vi "GetActionEventValue.vi"(8 "error in (no error)":errorcluster, 10 "Action":T1, 11 "WindowFrame in":refnum<class "WindowFrame.lvclass">) -> (0 "error out":errorcluster, 2 "Variant":variant, 3 "WindowFrame out":refnum<class "WindowFrame.lvclass">)   [LabVIEW 2021, in "WindowFrame.lvlib" / "WindowFrame.lvclass"]
uses:
  WindowFrame.lvclass
  Action.ctl
  ActionData.ctl
  GetEventActionRef.vi
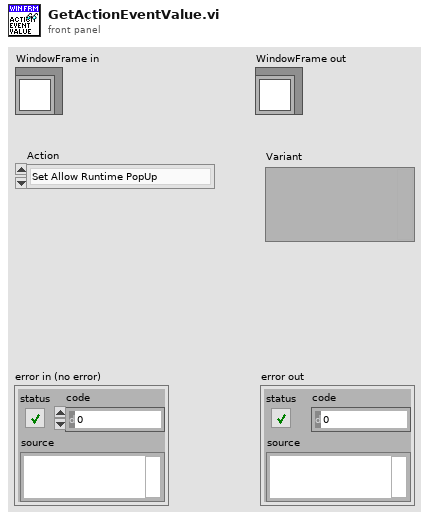
[diagram p1: front panel]
types:
  T1 = typedef "WindowFrame.lvlib/WindowFrame.lvclass/Action.ctl" = enum16{"Set Allow Runtime PopUp", "Set Behavior", "Set Closable", "Set Custom Title", "Set Highlight Return Button", "Set Is Frontmost", "Set Minimizable", "Set Minimum Size", "Set Monitor", "Set Resizable", "Set Panel Bounds", "Set Run VI Transparently", "Set Show Menu Bar", "Set State", "Set Title", "Set Title Bar Colors", "Set Title Bar Visible", "Set Transparancy", "Set Window Bounds", "Get Allow Runtime PopUp", "Get Behavior", "Get Closable", "Get Custom Title", "Get Highlight Return Button", "Get Is Frontmost", "Get Minimizable", "Get Minimum Size", "Get Monitor", "Get Panel Bounds", "Get Resizable", "Get Run VI Transparently", "Get Show Menu Bar", "Get State", "Get Title", "Get Title Bar Colors", "Get Title Bar Visible", "Get Transparancy", "Get Window Bounds", "--", "Center", "Close", "Open", "Run-Time Position:Centered", "Run-Time Position:Custom", "Run-Time Position:Get Position", "Run-Time Position:Maximized", "Run-Time Position:Minimized", "Run-Time Position:Unchanged", "---", "Insert VI", "Remove VI", "Insert VI Index", "Remove VI Index", "Exit"}
  T2 = typedef "WindowFrame.lvlib/WindowFrame.lvclass/ActionData.ctl" = cluster{"Action":T1, "Variant":variant}
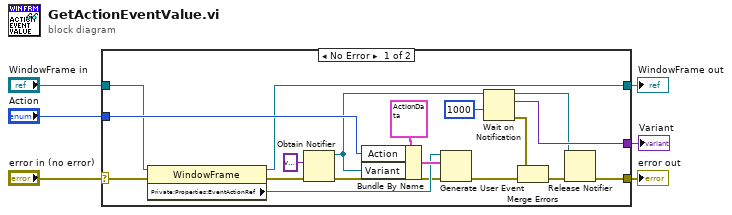
[diagram p0: block diagram]
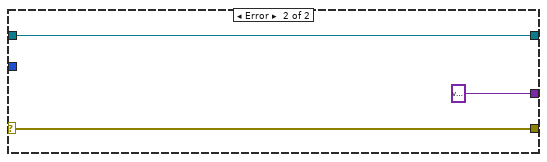
[diagram p2: hidden frame]
diagram:
  n1 = case shown="No Error" "error in (no error)" {
    selector: "error in (no error)" -> [w18 w26]
    tunnel: "Action" -> [w24 _]
    tunnel: [w8 w26] -> w5
    tunnel: "WindowFrame in" -> [w20 w27]
    tunnel: [w17 w27] -> w3
    tunnel: [w10 variant ("Variant")] -> w1
    frame No Error {
      n2 = property class="WindowFrame"(reference=w20, error in=w18) -> (reference out=w17:refnum<class "WindowFrame.lvclass">, error out=w16:errorcluster, "Private:Properties:EventActionRef"=w19:refnum<user-event>)
      n3 = Obtain Notifier(notification data type=variant ("Variant"), error in (no error)=w16) -> (notifier out=w11:refnum<notifier>, error out=w15:errorcluster)  [unwired: 2 in, 1 out]
      n4 = Bundle By Name(cluster=T2 {"Action"=enum."Set Allow Runtime PopUp", "Variant"=variant} ("event data"), "Action"=w24, "Variant"=w11) -> (w23:T2)
      n5 = Generate User Event(user event=w19, event data cluster=w23, error in=w15) -> (error out=w22:errorcluster)  [unwired: 1 in, 1 out]
      n6 = Wait on Notification(notifier=w11, timeout in ms (-1)=1000) -> (notifier out=w7:refnum<notifier>, notification=w10:variant, error out=w12:errorcluster)  [unwired: 2 in, 1 out]
      n7 = Merge Errors(w12, w22) -> (w13:errorcluster)
      n8 = Release Notifier(notifier=w7, error in (no error)=w13) -> (error out=w8:errorcluster)  [unwired: 1 in, 2 out]
    }
    frame Error {
    }
  }
  "error out" <- w5
  "WindowFrame out" <- w3
  "Variant" <- w1
